vi "Axial.vi"() -> ()   [LabVIEW 2017]
uses:
  <vilib>/Math Plots/2D Math Plots/XY Plot Matrix/XY Plot Matrix XCtrl/XY Plot Matrix.xctl
  <vilib>/Analysis/baseanly.llb/Mean (DBL).vi
  <vilib>/ULx/Create Channel.llb/ULx Create Channel (AI-Voltage-Basic).vi
  <vilib>/ULx/Timing.llb/ULx Timing (Sample Clock).vi
  <vilib>/ULx/Read.llb/ULx Read (Analog Wfm 1Chan NSamp).vi
  <vilib>/Math Plots/2D Math Plots/XY Plot Matrix/XY Plot Matrix Datatype/XY Plot Matrix Datatype.lvclass
  <vilib>/Analysis/NI_AALBase.lvlib
panel:
  out "Sample Button(Axial)":bool
  out "CalcRM":dbl[](array[numeric])
  out "CalcSF":dbl[](array[numeric])
  out "CalcPM":dbl[](array[numeric])
  out "CalcN":dbl[](array[numeric])
  out "CalcAxial":dbl[](array[numeric])
  out "CalcNormal":dbl[](array[numeric])
  in  "minimum value":dbl=-5.0
  in  "maximum value":dbl=5.0
  in  "samples per channel":i32=1000
  in  "sample mode":i32(ring) items=["FiniteSamples", "ContinuousSamples"]
  in  "rate":dbl=1000.0
  in  "Axial Force Physical Channel":refnum<k21>
  out "Voltage(R.M.)":dbl[](array[numeric])
  out "Voltage(S.F.)":dbl[](array[numeric])
  out "Voltage(P.M.)":dbl[](array[numeric])
  out "Voltage(n)":dbl[](array[numeric])
  out "Voltage(Normal)":dbl[](array[numeric])
  in  "Sample Button":bool
  out "Rolling Moment Plot":refnum<class "XY Plot Matrix Datatype.lvclass">[](xcontrol)
  out "S.F. Plot":refnum<class "XY Plot Matrix Datatype.lvclass">[](xcontrol)
  out "P.M. Plot":refnum<class "XY Plot Matrix Datatype.lvclass">[](xcontrol)
  out "n Plot":refnum<class "XY Plot Matrix Datatype.lvclass">[](xcontrol)
  out "Axial Force Plot":refnum<class "XY Plot Matrix Datatype.lvclass">[](xcontrol)
  out "Normal Force Plot":refnum<class "XY Plot Matrix Datatype.lvclass">[](xcontrol)
  out "Main Axial Force Plot":refnum<class "XY Plot Matrix Datatype.lvclass">[](xcontrol)
  in  "Add Weight":bool
  in  "Weight to be added":dbl
  out "Voltage(Axial)":dbl[](array[numeric])
  out "Weight":dbl[](array[numeric])
  out "Number of Data Cleared":dbl
  in  "Clear Table":bool
  # "Channel and Sampling Selection"
  # "Axial Force"
  # "Interaction Plots"
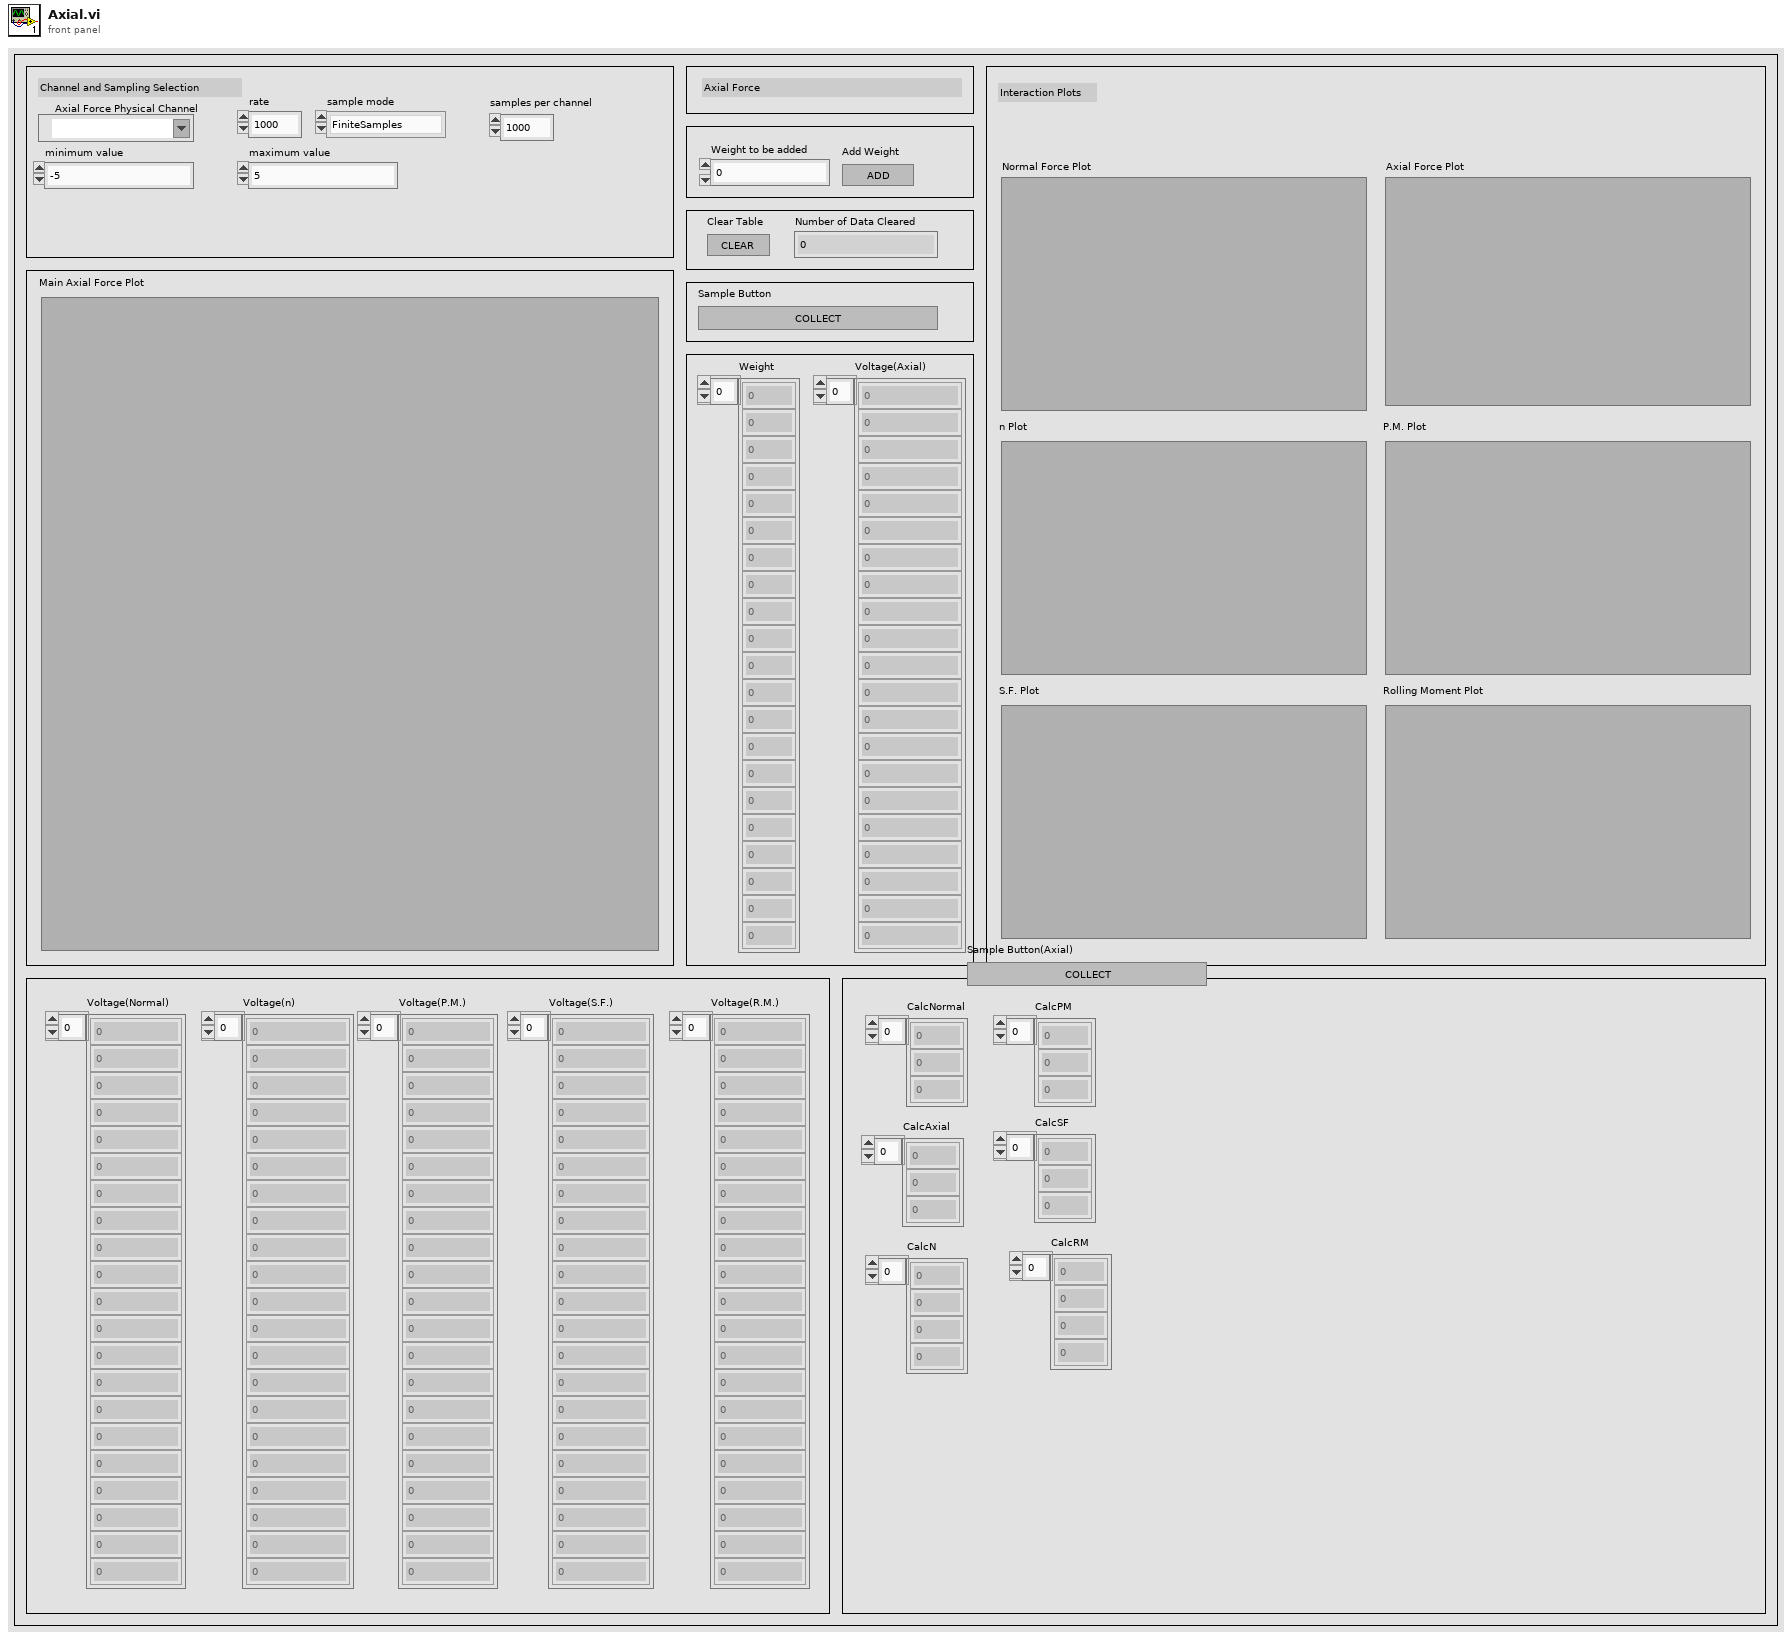
[diagram p1: front panel]
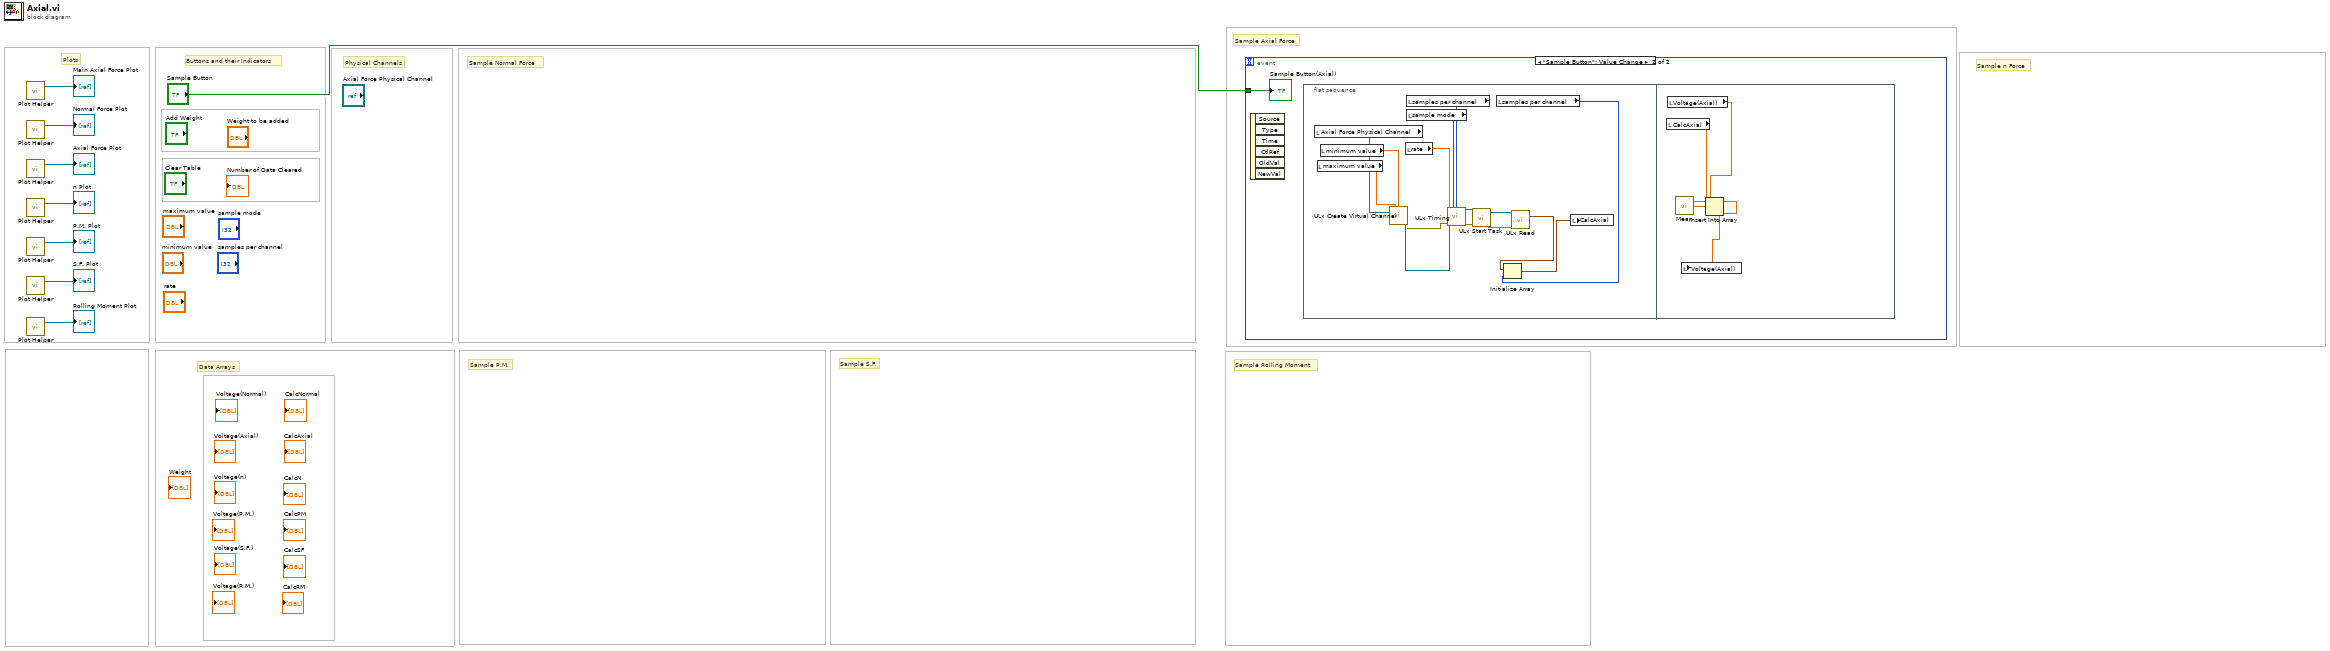
[diagram p0: block diagram]
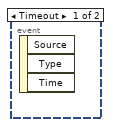
[diagram p2: hidden frame]
diagram:
  # "Physical Channels"
  # "Sample P.M."
  # "Sample Rolling Moment"
  # "Sample S.F."
  # "Sample n Force"
  # "Sample Axial Force"
  # "Sample Normal Force"
  # "Data Arrays"
  # "Buttons and their Indicators"
  # "Plots"
  n1 = call <vilib>:"Plot Helper.vi"() -> ("2D Plotmatrix Class Obj Array out"=→"Main Axial Force Plot":refnum<class "XY Plot Matrix Datatype.lvclass">[])  [unwired: 4 in, 7 out]
  n2 = call <vilib>:"Plot Helper.vi"() -> ("2D Plotmatrix Class Obj Array out"=→"Normal Force Plot":refnum<class "XY Plot Matrix Datatype.lvclass">[])  [unwired: 4 in, 7 out]
  n3 = call <vilib>:"Plot Helper.vi"() -> ("2D Plotmatrix Class Obj Array out"=→"Axial Force Plot":refnum<class "XY Plot Matrix Datatype.lvclass">[])  [unwired: 4 in, 7 out]
  n4 = call <vilib>:"Plot Helper.vi"() -> ("2D Plotmatrix Class Obj Array out"=→"n Plot":refnum<class "XY Plot Matrix Datatype.lvclass">[])  [unwired: 4 in, 7 out]
  n5 = call <vilib>:"Plot Helper.vi"() -> ("2D Plotmatrix Class Obj Array out"=→"P.M. Plot":refnum<class "XY Plot Matrix Datatype.lvclass">[])  [unwired: 4 in, 7 out]
  n6 = call <vilib>:"Plot Helper.vi"() -> ("2D Plotmatrix Class Obj Array out"=→"S.F. Plot":refnum<class "XY Plot Matrix Datatype.lvclass">[])  [unwired: 4 in, 7 out]
  n7 = call <vilib>:"Plot Helper.vi"() -> ("2D Plotmatrix Class Obj Array out"=→"Rolling Moment Plot":refnum<class "XY Plot Matrix Datatype.lvclass">[])  [unwired: 4 in, 7 out]
  n8 = event shown="[1] \"Sample Button\": Value Change" {
    selector: _ -> [_ _]
    dyn-events: _ -> [_ _]
    timeout: _ -> [_ _]
    tunnel: "Sample Button" -> [_ w9]
    event Timeout {
      n9 = event-data() -> ()  [unwired: 1 in, 3 out]
    }
    event "Sample Button": Value Change {
      n10 = event-data() -> ()  [unwired: 1 in, 6 out]
      n11 = flat-sequence {
        frame #0 {
          n12 = local read "Axial Force Physical Channel"() -> (w21:refnum<k21>)
          n13 = local read "maximum value"() -> (w17:dbl)
          n14 = local read "minimum value"() -> (w10:dbl)
          n15 = call-poly <vilib>:"ULx Create Virtual Channel.vi"("maximum value"=w17, "minimum value"=w10, "physical channels"=w21) -> ("task out"=w16:refnum<k24>, "error out"=w11:errorcluster)  [unwired: 11 in]
          n16 = local read "rate"() -> (w18:dbl)
          n17 = local read "samples per channel"() -> (w20:i32)
          n18 = local read "sample mode"() -> (w19:i32)
          n19 = call-poly <vilib>:"ULx Timing.vi"("task in"=w16, "sample mode"=w19, "samples per channel"=w20, "rate"=w18, "error in"=w11) -> ("task out"=w15:refnum<k24>, "error out"=w12:errorcluster)  [unwired: 9 in]
          n20 = call <vilib>:"ULx Start Task.vi"("task in"=w15, "error in"=w12) -> ("task out"=w14:refnum<k24>, "error out"=w13:errorcluster)  [unwired: 12 in]
          n21 = local read "samples per channel"() -> (w22:i32)
          n22 = call-poly <vilib>:"ULx Read.vi"("task in"=w14, "error in"=w13) -> ("data"=w23:waveform(dbl))  [unwired: 11 in, 2 out]
          n23 = Initialize Array(w23, w22) -> (w24:waveform(dbl)[])
          n24 = local write "CalcAxial"(w24) -> ()
        }
        frame #1 {
          n25 = local read "CalcAxial"() -> (w28:dbl[])
          n26 = local read "Voltage(Axial)"() -> (w27:dbl[])
          n27 = call-poly <vilib>:"Mean.vi"("X"=w28) -> ("mean"=w25:dbl)  [unwired: 1 out]
          n28 = Insert Into Array(array=w27, new element=w25) -> (w26:dbl[])  [unwired: 1 in]
          n29 = local write "Voltage(Axial)"(w26) -> ()
        }
      }
      "Sample Button(Axial)" <- w9
    }
  }
